vi "tablice.vi"() -> ()   [LabVIEW 2020]
uses:
  ebf3cfb9-b4de-4279-a918-55115f71fe46.vi
  <vilib>/Comparison/Less/Less Functor/Less Functor.lvclass
panel:
  out "Sorted":dbl[](array[numeric])
  in  "Last":dbl
  in  "First":dbl
  out "Subarray":dbl[](array[numeric])
  in  "stop":bool
  out "Scaled":dbl[](array[numeric])
  in  "Scale":dbl
  out "Random":dbl[](array[numeric])
  out "Numeric":dbl
  out "Gauge":dbl(knob) scale=0.0..10.0
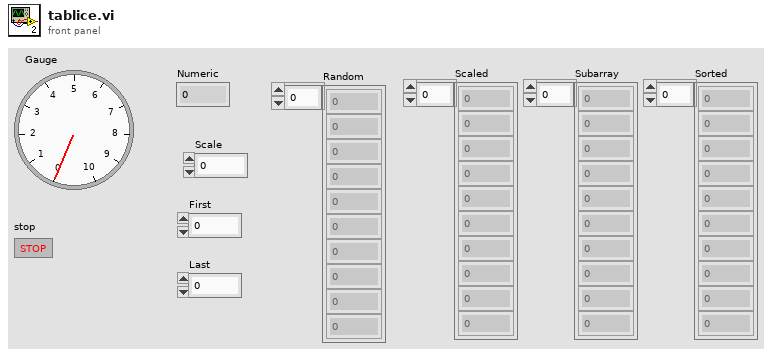
[diagram p1: front panel]
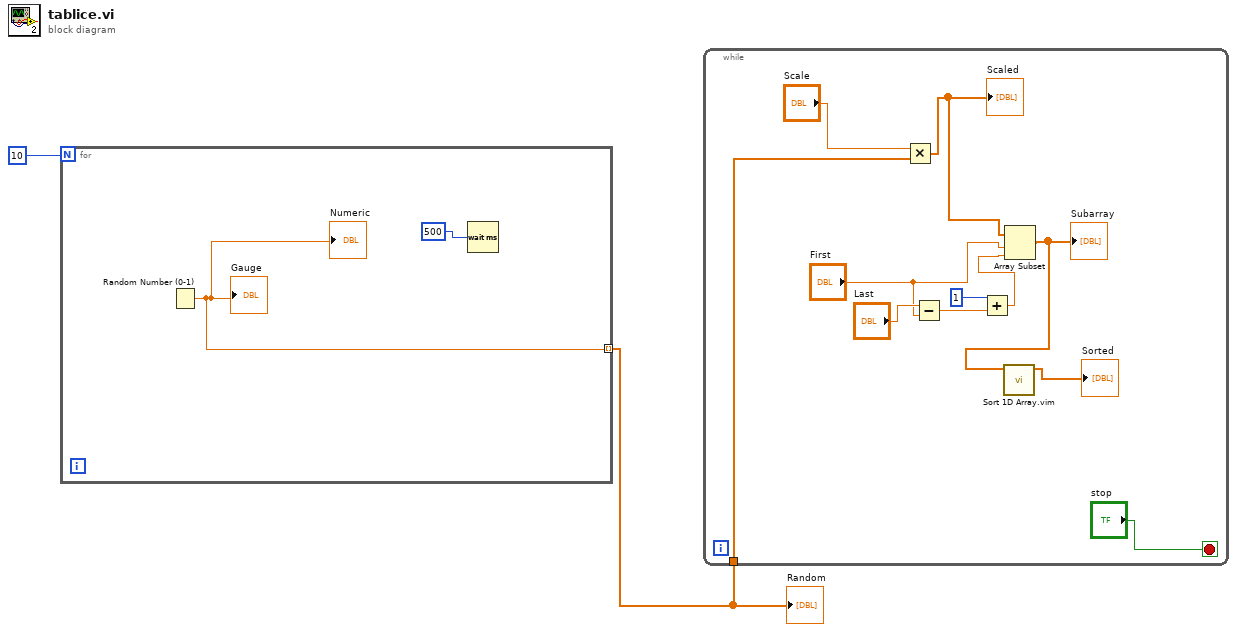
[diagram p0: block diagram]
diagram:
  n1 = for {
    N: 10 -> [_]
    tunnel: [w3] -> w1 mode=indexing
    n2 = Random Number (0-1)() -> (number: 0 to 1=w3:dbl)
    "Gauge" <- w3
    "Numeric" <- w3
    n3 = Wait (ms)(milliseconds to wait=500) -> ()  [unwired: 1 out]
  }
  "Random" <- w1
  n4 = while {
    tunnel: w1 -> [w10]
    stop <- "stop" stop-if-true
    n5 = Multiply(x="Scale", y=w10) -> (x*y=w5:dbl[])
    "Scaled" <- w5
    n6 = Subtract(x="Last", y="First") -> (x-y=w9:dbl)
    n7 = Add(x=1, y=w9) -> (x+y=w8:dbl)
    n8 = Array Subset(array=w5, index="First", length=w8) -> (w6:dbl[])
    "Subarray" <- w6
    n9 = call "Sort 1D Array.vim"("unsorted array"=w6) -> ("sorted array"=→"Sorted":dbl[])  [unwired: 10 in]
  }
